vi "Ini_file_RW_BoolGen.vi"(4 "Section":string="Init", 5 "Key":string="Key1", 6 "FileName":string="Config", 7 "Error in":errorcluster, 8 "FolderSource":T1(ring)=enum."Répertoire du parent 1" caption="SaveFolderSource", 9 "Write":bool, 10 "ValueIn":bool) -> (0 "Error out":errorcluster, 1 "file path":path caption="chemin du fichier", 3 "ValueOut":bool)   [LabVIEW 2019]
doc: "Ce VI ouvre le fichier de sauvegarde des modèles et lit les positions du modèle spécifié."
uses:
  <vilib>/Utility/config.llb/Read Key (Boolean).vi
  <vilib>/Utility/config.llb/Write Key (Boolean).vi
  <vilib>/Utility/config.llb/NI_LVConfig.lvlib
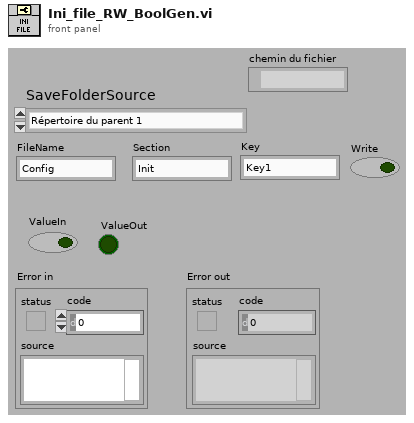
[diagram p1: front panel]
types:
  T1 = enum16{"Répertoire du VI actuel", "Répertoire du parent 1", "Répertoire du parent 2", "Répertoire du parent 3"}
  T2 = typedef "NI_LVConfig.lvlib/Config Data RefNum.ctl" = refnum<k1>
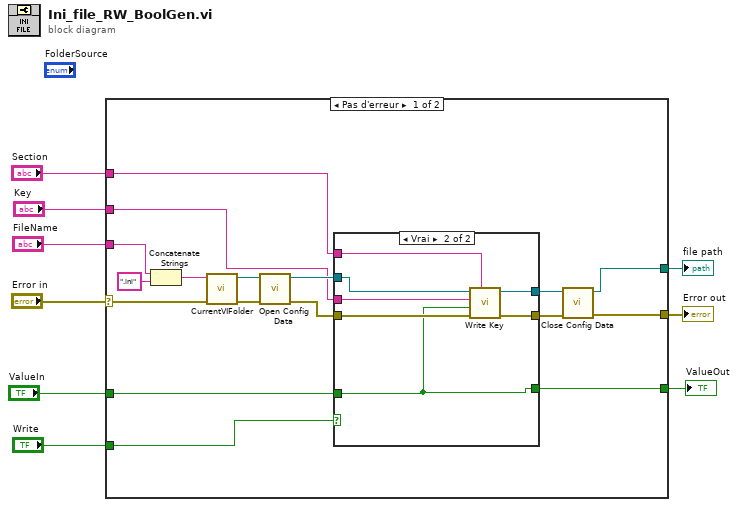
[diagram p0: block diagram]
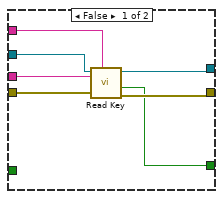
[diagram p2: hidden frame]
diagram:
  n1 = case shown="Pas d'erreur" "Error in" {
    selector: "Error in" -> [w21 w42]
    tunnel: [w20 w42] -> w9
    tunnel: "ValueIn" -> [w18 w41]
    tunnel: "Write" -> [w17 _]
    tunnel: [w16 w41] -> w5
    tunnel: "FileName" -> [w15 _]
    tunnel: "Key" -> [w12 _]
    tunnel: "Section" -> [w11 _]
    tunnel: [w10 _] -> w1
    frame No Error {
      n2 = Concatenate Strings(w15, ".ini" ("chaîne")) -> (w14:string)
      n3 = call <userlib>:"CurrentVIFolder.vi"("error in (no error)"=w21, "NomFichier"=w14) -> ("error out"=w26:errorcluster, "Chemin"=w19:path)  [unwired: 7 in, 1 out]
      n4 = call <vilib>:"Open Config Data.vi"("error in (no error)"=w26, "configuration file path"=w19) -> ("error out"=w23:errorcluster, "refnum"=w25:T2)  [unwired: 7 in, 1 out]
      n5 = case shown="Vrai" w17 {
        tunnel: w25 -> [w30 w36]
        tunnel: w11 -> [w32 w40]
        tunnel: [w29 w39] -> w24
        tunnel: w23 -> [w33 w38]
        tunnel: [w28 w37] -> w22
        tunnel: w18 -> [_ w34]
        tunnel: w12 -> [w31 w35]
        tunnel: [w27 w34] -> w16
        frame False {
          n6 = call-poly <vilib>:"Read Key.vi"("section"=w32, "error in (no error)"=w33, "key"=w31, "refnum"=w30) -> ("error out"=w28:errorcluster, "value"=w27:bool, "refnum out"=w29:T2)  [unwired: 4 in, 1 out]
        }
        frame True {
          n7 = call-poly <vilib>:"Write Key.vi"("section"=w40, "error in (no error)"=w38, "value"=w34, "key"=w35, "refnum"=w36) -> ("error out"=w37:errorcluster, "refnum out"=w39:T2)  [unwired: 4 in, 1 out]
        }
      }
      n8 = call <vilib>:"Close Config Data.vi"("error in (no error)"=w22, "refnum"=w24) -> ("error out"=w20:errorcluster, "file path"=w10:path)  [unwired: 8 in]
    }
    frame Error {
    }
  }
  "Error out" <- w9
  "ValueOut" <- w5
  "file path" <- w1
